vi "CloseGlobalPanels.vi"   [LabVIEW 2019]
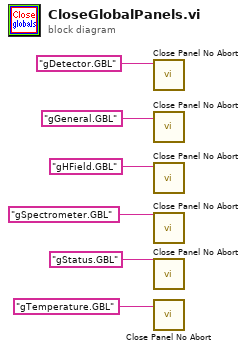
[diagram p0: block diagram]
diagram:
  n1 = call <vilib>:"Close Panel No Abort.vi"("VI name"="gDetector.GBL" ("name or relative path")) -> ()  [unwired: 10 in, 1 out]
  n2 = call <vilib>:"Close Panel No Abort.vi"("VI name"="gGeneral.GBL" ("name or relative path")) -> ()  [unwired: 10 in, 1 out]
  n3 = call <vilib>:"Close Panel No Abort.vi"("VI name"="gHField.GBL" ("name or relative path")) -> ()  [unwired: 10 in, 1 out]
  n4 = call <vilib>:"Close Panel No Abort.vi"("VI name"="gSpectrometer.GBL" ("name or relative path")) -> ()  [unwired: 10 in, 1 out]
  n5 = call <vilib>:"Close Panel No Abort.vi"("VI name"="gStatus.GBL" ("name or relative path")) -> ()  [unwired: 10 in, 1 out]
  n6 = call <vilib>:"Close Panel No Abort.vi"("VI name"="gTemperature.GBL" ("name or relative path")) -> ()  [unwired: 10 in, 1 out]
